vi "close.vi"(8 "error in (no error)":errorcluster, 11 "Compiler in":refnum<class "Compiler.lvclass">) -> (0 "error out":errorcluster, 3 "Compiler out":refnum<class "Compiler.lvclass">)   [LabVIEW 2009, in "Compiler.lvlib" / "Compiler.lvclass"]
uses:
  Compiler.lvclass
  Compiler.lvclass/Compiler.ctl
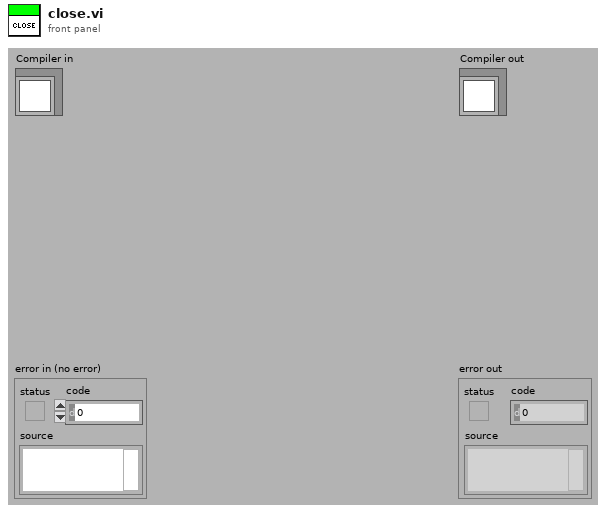
[diagram p1: front panel]
types:
  T1 = enum32{"Bad", "Idle", "Run top level", "Running"}
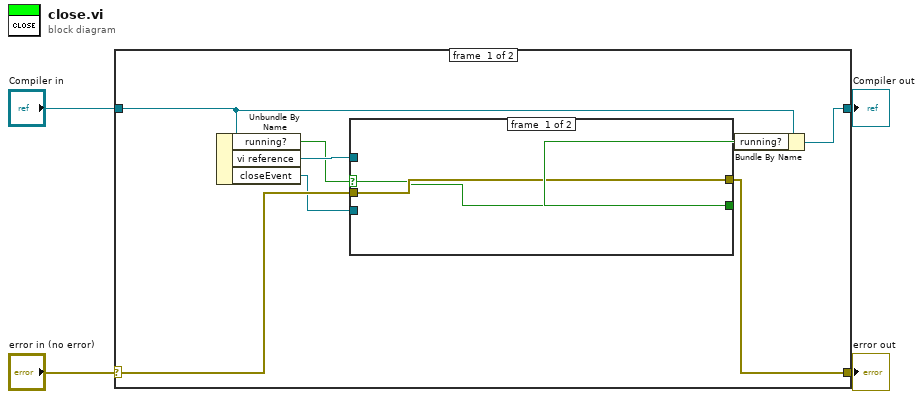
[diagram p0: block diagram]
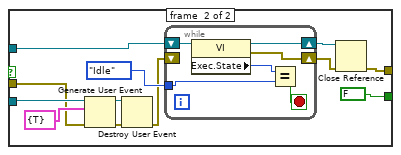
[diagram p2: hidden frame]
diagram:
  n1 = case shown="No Error" "error in (no error)" {
    selector: "error in (no error)" -> [w10 w34]
    tunnel: [w9 w34] -> w1
    tunnel: [w6 w33] -> w2
    tunnel: "Compiler in" -> [w7 w33]
    frame #0 {
      n2 = Unbundle By Name(w7) -> ("running?"=w11:bool, "vi reference"=w12:refnum<vi>, "closeEvent"=w5:refnum<user-event>)
      n3 = case shown="True" w11 {
        selector: w11 -> [w13 _]
        tunnel: w12 -> [_ w20]
        tunnel: w10 -> [w14 w19]
        tunnel: [w14 w26] -> w9
        tunnel: [w13 FALSE] -> w8
        tunnel: w5 -> [_ w24]
        frame #0 {
        }
        frame #1 {
          n4 = Generate User Event(user event=w24, event data cluster=cluster{"close":bool} {"close"=TRUE} ("event data"), error in=w19) -> (user event out=w16:refnum<user-event>, error out=w17:errorcluster)
          n5 = Destroy User Event(user event=w16, error in=w17) -> (error out=w15:errorcluster)
          n6 = while {
            shift-right: [w31] -> w21
            shift-left: w15 -> [_]
            shift-right: [w32] -> w22
            shift-left: w20 -> [w30]
            tunnel: T1."Idle" ("Execution:State") -> [w28]
            stop <- w27 stop-if-true
            n7 = property class="VI"(reference=w30) -> (reference out=w32:refnum<vi>, error out=w31:errorcluster, "Exec.State"=w29:T1)  [unwired: 1 in]
            n8 = Equal?(x=w29, y=w28) -> (x = y?=w27:bool)
          }
          n9 = Close Reference(reference=w22, error in (no error)=w21) -> (error out=w26:errorcluster)
        }
      }
      n10 = Bundle By Name(cluster=w7, "running?"=w8) -> (w6:refnum<class "Compiler.lvclass">)
    }
    frame #1 {
    }
  }
  "error out" <- w1
  "Compiler out" <- w2
